vi "Client RX Loop.vi"(8 "error in (no error)":errorcluster, 11 "TCPMessaging in":refnum<class "TCPMessaging.lvclass">) -> (0 "error out":errorcluster)   [LabVIEW 2020, in "Vecto.lvlib" / "TCPMessaging.lvclass"]
uses:
  TCPMessaging.lvclass
  TCPMessaging.lvclass/TCPMessaging.ctl
  EventLoggingService/EventLoggingService.lvclass/EventLoggingService.ctl
  <vilib>/Utility/error.llb/Error Cluster From Error Code.vi
  EventLogHandler/EventLogHandler.lvclass
  EventLoggingService/EventLoggingService.lvclass
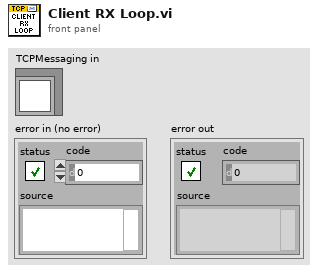
[diagram p1: front panel]
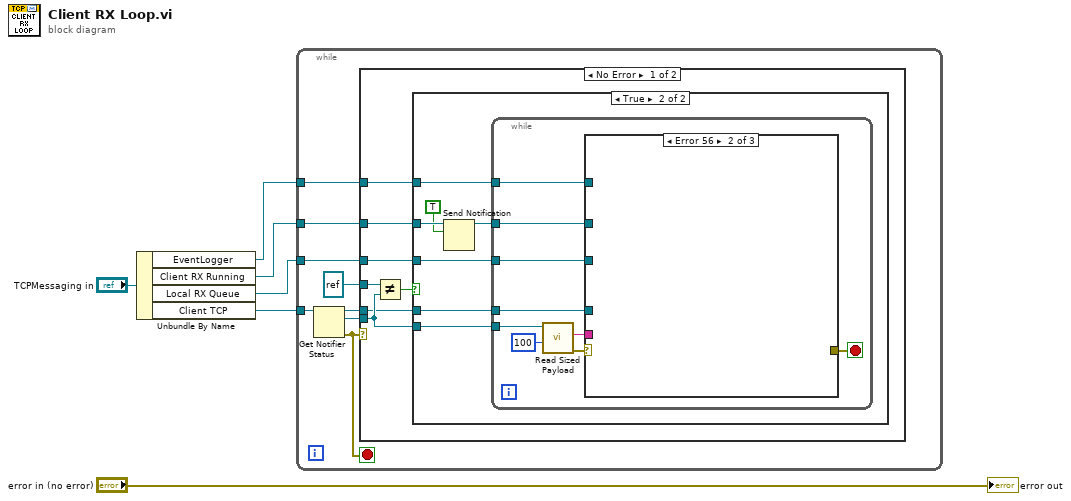
[diagram p0: block diagram]
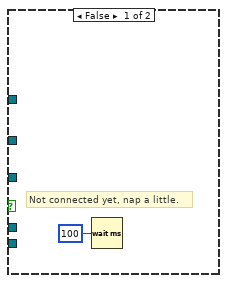
[diagram p2: hidden frame]
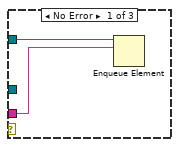
[diagram p3: hidden frame]
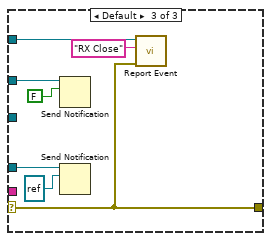
[diagram p4: hidden frame]
diagram:
  n1 = Unbundle By Name("TCPMessaging in") -> ("EventLogger"=w1:refnum<class "EventLoggingService.lvclass">, "Client RX Running"=w2:refnum<notifier>, "Local RX Queue"=w3:refnum<queue>, "Client TCP"=w4:refnum<notifier>)
  n2 = while {
    tunnel: w4 -> [w14]
    tunnel: w3 -> [w10]
    tunnel: w2 -> [w9]
    tunnel: w1 -> [w7]
    stop <- w12 stop-if-true
    n3 = Get Notifier Status(notifier=w14) -> (notifier out=w8:refnum<notifier>, current notification=w13:refnum<k5>, error out=w12:errorcluster)  [unwired: 1 in, 2 out]
    n4 = case shown="No Error" w12 {
      tunnel: w13 -> [w19 _]
      tunnel: refnum<k5> refnum ("x") -> [w21 _]
      tunnel: w10 -> [w18 _]
      tunnel: w9 -> [w17 _]
      tunnel: w8 -> [w16 _]
      tunnel: w7 -> [w15 _]
      frame No Error {
        n5 = Not Equal?(x=w21, y=w19) -> (x != y?=w20:bool)
        n6 = case shown="True" w20 {
          tunnel: w19 -> [_ w29]
          tunnel: w18 -> [_ w28]
          tunnel: w17 -> [_ w27]
          tunnel: w16 -> [_ w24]
          tunnel: w15 -> [_ w23]
          frame False {
            # "Not connected yet, nap a little."
            n7 = Wait (ms)(milliseconds to wait=u32 100) -> ()  [unwired: 1 out]
          }
          frame True {
            n8 = Send Notification(notification=TRUE, notifier=w27) -> (notifier out=w26:refnum<notifier>)  [unwired: 1 in, 1 out]
            n9 = while {
              tunnel: w29 -> [w37]
              tunnel: w28 -> [w38]
              tunnel: w26 -> [w32]
              tunnel: w24 -> [w31]
              tunnel: w23 -> [w30]
              stop <- w33 stop-if-true
              n10 = call "Read Sized Payload.vi"("timeout ms (100)"=100, "TCP in"=w37) -> ("error out"=w35:errorcluster, "Payload"=w34:string)  [unwired: 7 in, 1 out]
              n11 = case shown="Error 56" w35 {
                selector: w35 -> [_ _ w41]
                tunnel: w38 -> [w40 _ _]
                tunnel: w34 -> [w39 _ _]
                tunnel: [_ _ w41] -> w33
                tunnel: w32 -> [_ _ w47]
                tunnel: w31 -> [_ _ w45]
                tunnel: w30 -> [_ _ w43]
                frame No Error {
                  n12 = Enqueue Element(queue=w40, element=w39) -> ()  [unwired: 2 in, 3 out]
                }
                frame Error {
                }
                frame Default {
                  n13 = Send Notification(notification=FALSE, notifier=w47) -> ()  [unwired: 1 in, 2 out]
                  n14 = Send Notification(notification=refnum<k5> refnum, notifier=w45) -> ()  [unwired: 1 in, 2 out]
                  n15 = call "Report Event.vi"("error in (no error)"=w41, "Message"="RX Close", "EventLoggingService in"=w43) -> ()  [unwired: 7 in, 2 out]
                }
              }
            }
          }
        }
      }
      frame Error {
        # "Notifier has been released, shutting down."
      }
    }
  }
  "error out" <- "error in (no error)"
